vi "模拟器自动控制程序（轨迹跟踪）[2.1 alpha].vi"() -> ()   [LabVIEW 2012]
uses:
  <vilib>/Utility/error.llb/DialogType.ctl
  <vilib>/Platform/TimedLoop/XDataNode/timing_clust.ctl
  <vilib>/Platform/TimedLoop/XDataNode/nitl_modes.ctl
  <vilib>/Platform/TimedLoop/XDataNode/wakeup.ctl
  <vilib>/Instr/_visa.llb/VISA Configure Serial Port (Instr).vi
  <vilib>/DAQmx/create/channels.llb/DAQmx Create Channel (DO-Digital Output).vi
  <vilib>/Analysis/baseanly.llb/Real Dot Product.vi
  <vilib>/Analysis/Matrix/Numeric/Conversions/Array To Matrix - RA2.vi
  <vilib>/Utility/file.llb/Write To Spreadsheet File (DBL).vi
  <vilib>/Platform/TimedLoop/XDataNode/XDataNode.xnode
  <vilib>/Platform/TimedLoop/XDataNode/XDNodeRunTimeDep.lvlib
  <vilib>/Analysis/Matrix/NI_Matrix.lvlib
  <vilib>/vision/NI_Vision_Development_Module.lvlib
  <vilib>/Analysis/NI_AALBase.lvlib
panel:
  out "x/y":dbl
  out "Truster4":bool
  out "Truster 8":bool
  out "Truster  3":bool
  out "Truster 7":bool
  out "Truster 5":bool
  out "Truster  2":bool
  out "Truster 6":bool
  out "Truster1":bool
  out "定位点信息":T1(array[cluster]) {"Aspect Ratio" format="%.2f"; "Orientation" format="%.2f"; "Area" format="%.2f"; "Object Center"."Y" format="%.2f"; "Object Center"."X" format="%.2f"}
  out "alpha":dbl
  out "计时参数":dbl
  in  "卫星模拟器":enum32{"初始化", "运行监测"}(tab)
  out "读取缓冲区":string
  out "电流校正模式":bool
  out "软件使能":bool caption="软件使能(启动/停止)"
  out "电流校正中":bool caption="电流校正完成"
  out "E2PROM初始化结果":bool
  out "E2初始化完成":bool
  out "CRC校验和错误":bool
  out "串口通信错误":bool caption="串口通信故障"
  out "发送指令":string
  out "控制命令":string
  out "电机已启动":bool
  in  "采样率":i64=10
  in  "限制转速":dbl=500.0
  in  "ID号":u8=255 step=1 format="%#.0f"
  in  "最高转速":dbl=500.0
  in  "PWM周期":dbl=1599.0
  in  "最大力矩":dbl=2047.0
  in  "stop bits (10: 1 bit)":u16(ring)=10 caption="停止位" items=["1.0"=10, "1.5"=15, "2.0"=20]
  out "串口状态":bool
  in  "端口选择":refnum<visa-resource-name>="COM1"
  in  "波特率":u16(ring)=10 items=["   300", "   600", "   1200", "   2400", "   4800   ", "   9600", "   19200", "   38400", "   43000", "   56000", "   57600", "   115200"]
  in  "校验":enum16{"None", "Odd", "Even"}(ring)=enum."Even"
  in  "数据位":u16=8
  in  "打开":bool caption="stop"
  out "轨控信号":dbl
  in  "姿轨控开始":bool
  out "转速模式":bool
  out "转矩模式":bool
  out "故障":bool
  out "启停状态":bool
  in  "存储波形":bool
  in  "显示波形 停止显示":bool
  in  "开始记录":bool
  out "动量轮转矩":dbl format="%#_6f"
  out "动量轮转速":dbl format="%#_4f"
  out "X速率(cm/s)":dbl
  out "Y速率(cm/s)":dbl
  out "Y偏移量 (cm)":dbl
  out "X偏移量 (cm)":dbl
  out "相对偏角(deg)":dbl
  out "角速度(deg/s)":dbl
  out "设备ID":u8=255
  in  "模式选择":u16(ring)=1 items=["电流校正模式", "转矩模式", "转速模式", "开环测试模式"]
  in  "模式选择":bool
  in  "写指令字":dbl
  in  "清除故障":bool
  in  "停止电机":bool
  in  "启动电机":bool
  out "波形图":cluster{"转矩反馈":dbl, "转速反馈":dbl}(graph)
  in  "退出程序":bool caption="停止电机 2"
  in  "Floating":bool
  in  "缩放比例 (像素/cm)":dbl=4.099468
  in  "X中心校正":dbl
  in  "Y中心校正":dbl
  out "指令Y":dbl
  out "指令X":dbl
  out "指令角度":dbl
  out "alpha (deg)":dbl
  out "x >= y?":bool
  out "数值":dbl
  out "输出数组 6":dbl[](array[numeric])
  out "输出数组 7":dbl[](array[numeric])
  out "输出数组 10":dbl[](array[numeric])
  out "无符号字节数组 2":u8[](array[numeric])
  # "状态"
  # "设置"
  # "控制信号"
  # "参数确定"
  # "状态显示"
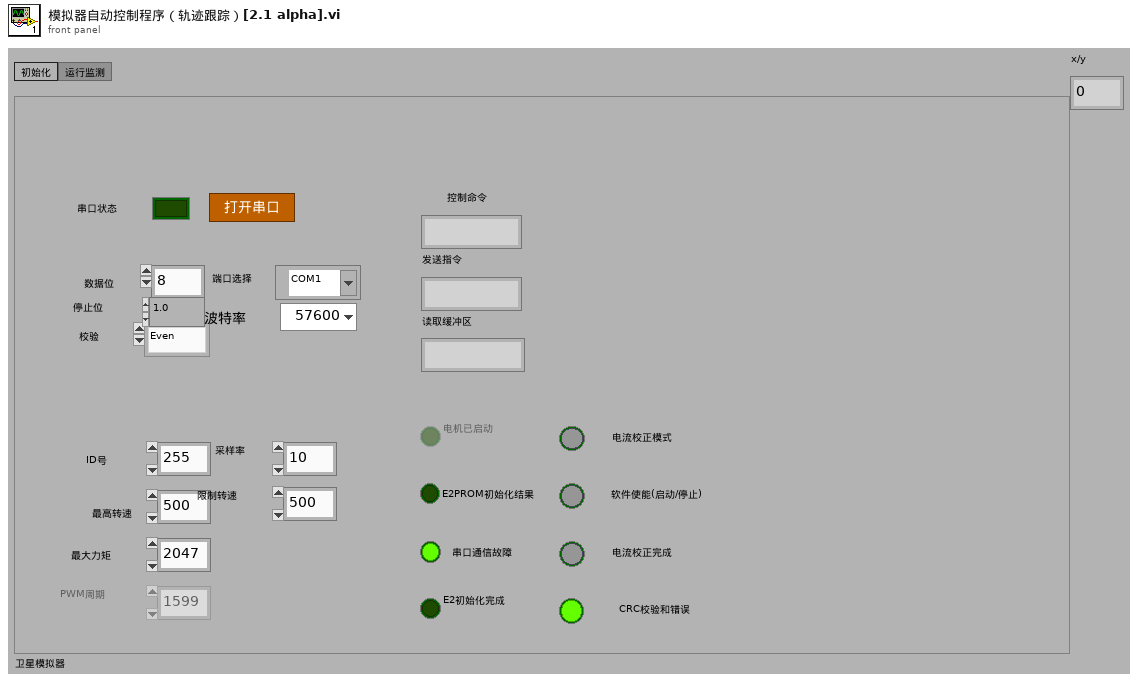
[diagram p1: front panel]
types:
  T1 = cluster{"Object Center":cluster{"X":sgl, "Y":sgl}, "Bounding Box":cluster{"X Left":i32, "Y Top":i32, "X Right":i32, "Y Bottom":i32}, "Area":sgl, "Orientation":sgl, "Aspect Ratio":sgl, "Nb Holes":i32}[]
  T2 = typedef "XDNodeRunTimeDep.lvlib/timing_clust.ctl" = cluster{"Expected End [f-1]":u64, "Actual End [f-1]":u64, "Finished Late? [f-1]":bool, "Expected End [i-1]":u64, "Actual End [i-1]":u64, "Finished Late? [i-1]":bool, "Expected Start [i]":u64, "Actual Start [i]":u64, "Expected Start [f]":u64, "Actual Start [f]":u64, "Source Name":string, "Structure Name":string, "Period":i64, "Deadline":i64, "Offset":i64, "Start":i64, "Priority":i32, "Timeout":i32, "Mode":T3, "Wakeup Reason":T4, "Error":errorcluster, "Source Type":string, "Secondary Source Type":string, "Global End Time":u64, "Global Start Time":u64, "Frame Duration":u64, "Iteration Duration":u64, "Assigned CPU":i32, "I/O Scan Engine Mode":u32}
  T3 = typedef "XDNodeRunTimeDep.lvlib/nitl_modes.ctl" = enum32{"No Change", "Process missed periods, maintain original phase", "Discard missed periods, maintain original phase", "Process missed periods, ignore original phase", "Discard missed periods, ignore original phase"}
  T4 = typedef "XDNodeRunTimeDep.lvlib/wakeup.ctl" = enum32{"Normal", "Aborted", "Asynchronous wakeup", "Timing source error", "Timed loop error", "Timeout"}
  T5 = cluster{"Objects":u16, "Threshold":i32, "Reject Border":bool, "Fill Holes":bool, "Min Object Size":bool, "Min Size":i32, "Max Object Size":bool, "Max Size":i32, "Show Search Area":bool, "Show Center":bool, "Show Bounding Box":bool}
  T6 = typedef "DialogType.ctl" = u16
  T7 = typedef "NI_Matrix.lvlib/RealMatrix.ctl" = dbl[][]
  T8 = typedef "IMAQ Image.ctl" = refnum<image>
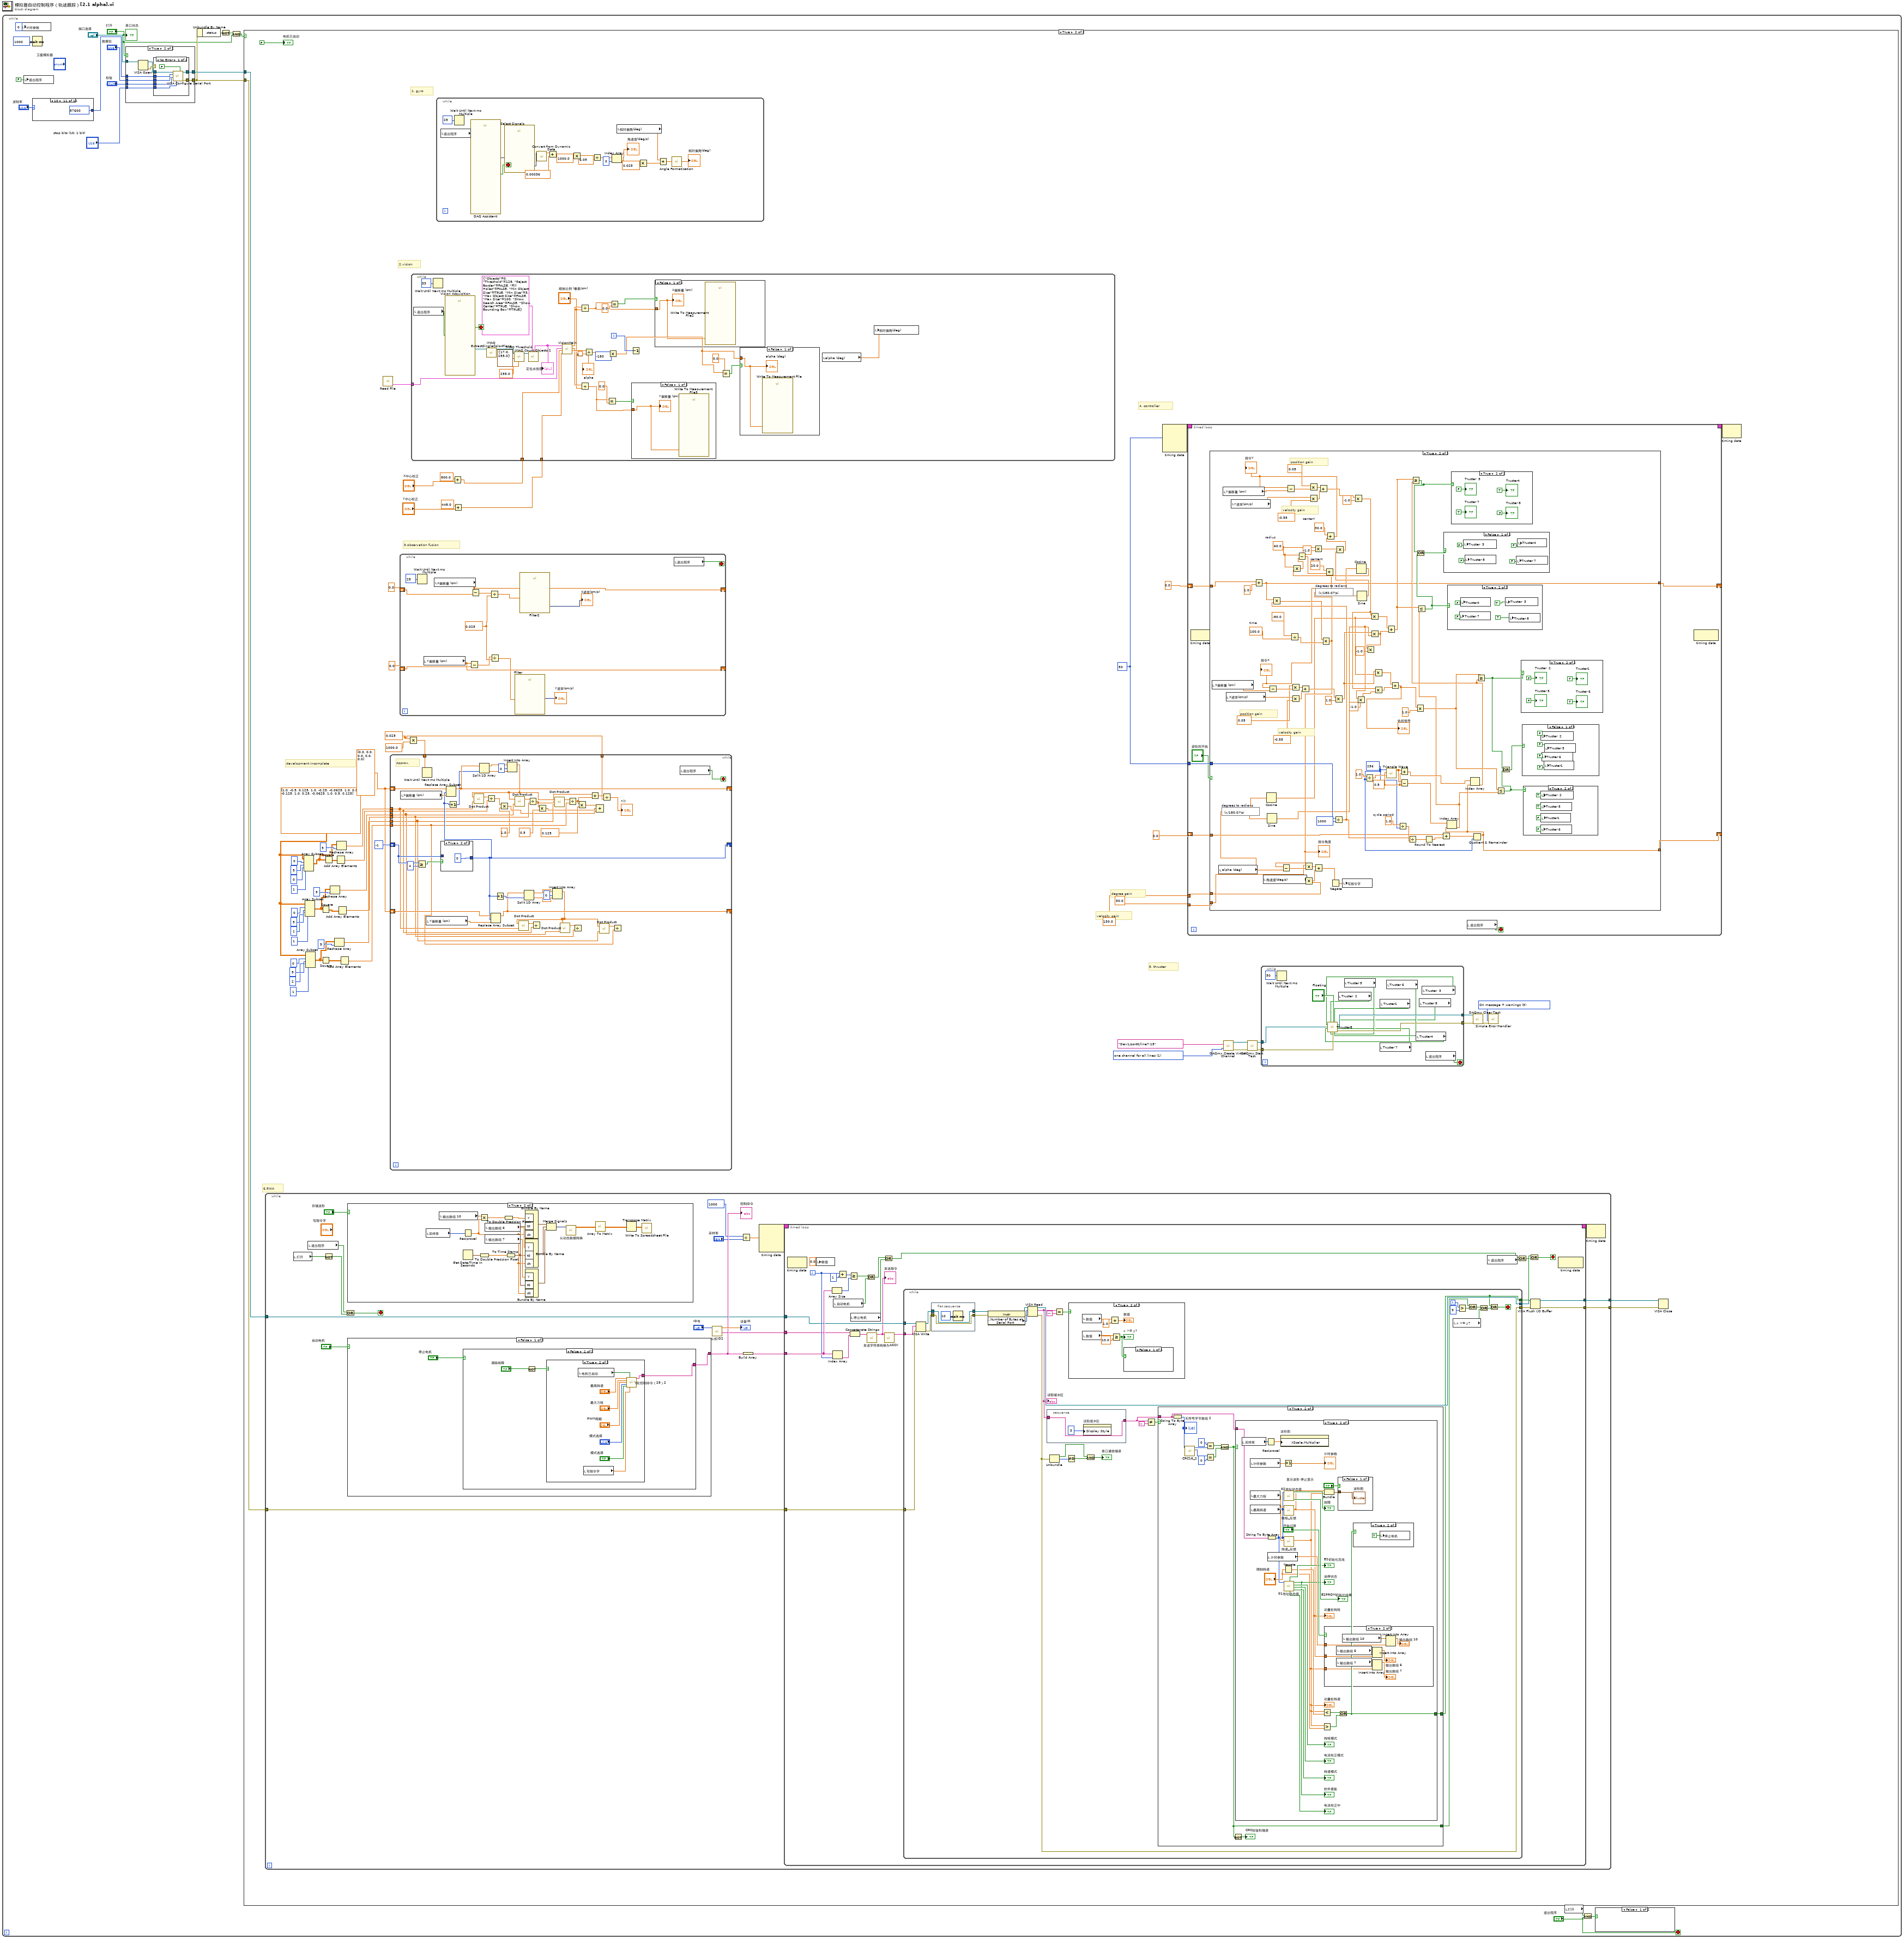
[diagram p0: block diagram]
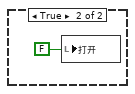
[diagram p2: hidden frame]
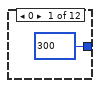
[diagram p5: hidden frame]
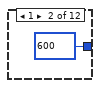
[diagram p6: hidden frame]
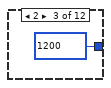
[diagram p7: hidden frame]
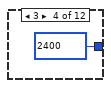
[diagram p8: hidden frame]
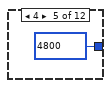
[diagram p9: hidden frame]
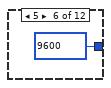
[diagram p10: hidden frame]
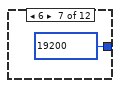
[diagram p11: hidden frame]
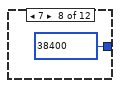
[diagram p12: hidden frame]
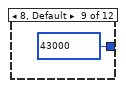
[diagram p13: hidden frame]
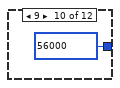
[diagram p14: hidden frame]
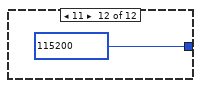
[diagram p15: hidden frame]
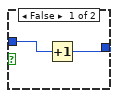
[diagram p17: hidden frame]
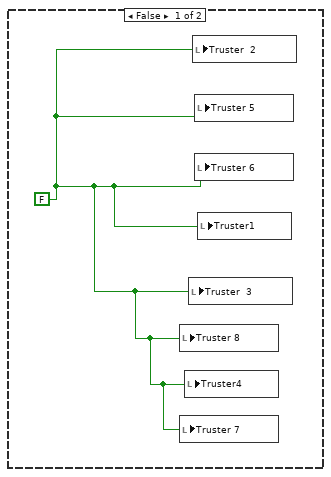
[diagram p18: hidden frame]
diagram:
  n1 = while {
    stop <- "退出程序" stop-if-true
    n2 = local write "计时参数"(0) -> ()
    n3 = local write "退出程序"(FALSE ("退出程序")) -> ()
    n4 = Wait (ms)(milliseconds to wait=u32 1000 ("等待时间（毫秒）")) -> ()  [unwired: 1 out]
    n5 = case shown="10" "波特率" {
      tunnel: [300 600 1200 2400 4800 9600 19200 38400 43000 56000 57600 115200] -> w17
      frame 0 {
      }
      frame 1 {
      }
      frame 2 {
      }
      frame 3 {
      }
      frame 4 {
      }
      frame 5 {
      }
      frame 6 {
      }
      frame 7 {
      }
      frame 8, Default {
      }
      frame 9 {
      }
      frame 10 {
      }
      frame 11 {
      }
    }
    n6 = case shown="True" "打开" {
      tunnel: w17 -> [_ w28]
      tunnel: "数据位" -> [_ w27]
      tunnel: "校验" -> [_ w26]
      tunnel: "端口选择" -> [_ w25]
      tunnel: [_ w22] -> w7
      tunnel: [_ w21] -> w6
      tunnel: "stop bits (10: 1 bit)" -> [_ w20]
      frame False {
      }
      frame True {
        n7 = VISA Open(VISA resource name=w25) -> (VISA resource name=w24:refnum<visa-resource-name>, error out=w23:errorcluster)  [unwired: 1 in, 3 out]
        n8 = case shown="No Error" w23 {
          tunnel: w28 -> [w36 _]
          tunnel: w27 -> [w35 _]
          tunnel: w26 -> [w34 _]
          tunnel: w24 -> [w33 _]
          tunnel: [w32 _] -> w22
          tunnel: [w31 _] -> w21
          tunnel: w20 -> [w30 _]
          frame No Error {
            n9 = call-poly "VISA Configure Serial Port"("VISA resource name"=w33, "Enable Termination\nChar (T)"=FALSE ("Enable Termination\nChar (T)"), "baud rate (9600)"=w36, "data bits (8)"=w35, "parity (0:none)"=w34, "stop bits (10: 1 bit)"=w30) -> ("VISA resource name out"=w32:refnum<visa-resource-name>, "error out"=w31:errorcluster)  [unwired: 2 in, 6 out]
          }
          frame Error {
          }
        }
      }
    }
    n10 = Unbundle By Name(w6) -> ("status"=w12:bool)
    n11 = Not(x=w12) -> (.not. x?=w11:bool)
    n12 = And(x=w11, y="打开") -> (x .and. y?=w8:bool)
    n13 = case shown="True" w8 {
      tunnel: w7 -> [_ w109]
      tunnel: w6 -> [_ w108]
      frame False {
      }
      frame True {
        w49 = 0.025
        w65 = dbl[][] [[1.0, -0.5, 0.125], [1.0, -0.25, -0.0625], [1.0, 0.0, -0.125], [1.0, 0.25, -0.0625], [1.0, 0.5, 0.125]]
        w52 = dbl[] [0.0, 0.0, 0.0, 0.0, 0.0]
        w89 = 1 items=["one channel for each line", "one channel for all lines"] ("line grouping")
        w91 = T6 3 items=["no dialog", "OK message", "continue or stop message", "OK message + warnings", "continue/stop + warnings"] ("type of dialog (OK msg:1)")
        w85 = 50
        # "development incomplete"
        # "5. thruster"
        # "6.RWA"
        # "4. controller"
        # "3.observation fusion"
        # "2.vision"
        # "1. gyro"
        # "velocity gain"
        # "degree gain"
        n14 = while {
          tunnel: [w379] -> w111
          tunnel: [w378] -> w110
          tunnel: w109 -> [w377]
          tunnel: w108 -> [w376]
          stop <- w372 stop-if-true
          n15 = local read "打开"() -> (w375:bool)
          n16 = local read "退出程序"() -> (w374:bool)
          n17 = Not(x=w375) -> (.not. x?=w373:bool)
          n18 = Or(x=w374, y=w373) -> (x .or. y?=w372:bool)
          n19 = case shown="True" "存储波形" {
            frame False {
            }
            frame True {
              n20 = local read "采样率"() -> (w404:i64)
              n21 = local read "输出数组 10"() -> (w397:dbl[])
              n22 = Reciprocal(x=w404) -> (1/x=w399:dbl)
              n23 = Get Date/Time In Seconds() -> (seconds since 1Jan1904=w408:timestamp)
              n24 = Multiply(x=w397, y=w399) -> (x*y=w398:dbl[])
              n25 = To Double Precision Float(number=w408) -> (double precision float=w407:dbl)
              n26 = local read "输出数组 6"() -> (w406:dbl[])
              n27 = local read "输出数组 7"() -> (w405:dbl[])
              n28 = To Double Precision Float(number=w398) -> (double precision float=w396:dbl[])
              n29 = To Time Stamp(1:w407) -> (0:w400:timestamp)
              n30 = Bundle By Name("Y"=w396, "t0"=w400, "dt"=w399) -> (w401:waveform(dbl))  [unwired: 1 out]
              n31 = Bundle By Name("Y"=w406, "t0"=w400, "dt"=w399) -> (w402:waveform(dbl))  [unwired: 1 out]
              n32 = Bundle By Name("Y"=w405, "t0"=w400, "dt"=w399) -> (w403:waveform(dbl))  [unwired: 1 out]
              n33 = Merge Signals(w401, w402, w403) -> (w395:dynamicdata)
              n34 = call "从动态数据转换"("Dynamic Data Type"=w395) -> ("Array"=w394:dbl[][])  [unwired: 3 in]
              n35 = call-poly <vilib>:"Array To Matrix.vi"("Real 2D Array"=w394) -> ("Real Matrix"=w393:T7)
              n36 = Transpose Matrix(1:w393) -> (0:w392:T7)
              n37 = call-poly <vilib>:"Write To Spreadsheet File.vi"("2D data"=w392) -> ()  [unwired: 7 in, 1 out]
            }
          }
          n38 = case shown="False" "启动电机" {
            tunnel: [w535 w562] -> w388
            frame False {
              n39 = case shown="False" "停止电机" {
                tunnel: [w536 w555] -> w535
                frame False {
                  n40 = Not(x="清除故障") -> (.not. x?=w537:bool)
                  n41 = case shown="True" w537 {
                    tunnel: [w539 w548] -> w536
                    frame False {
                      n42 = call <vilib>:"Space Constant.vi"() -> ("String"=w543:string)
                      n43 = Concatenate Strings(w543, "05" ("字符串"), w543, "23" ("字符串"), w543, "01" ("字符串")) -> (w539:string)
                    }
                    frame True {
                      n44 = local read "电机已启动"() -> (w545:bool)
                      n45 = local read "写指令字"() -> (w544:dbl)
                      n46 = call "飞轮控制命令（29）2.vi"("最高转速"="最高转速", "电机启动控制指令"=w545, "力矩最大值"="最大力矩", "pwmperiod"="PWM周期", "模式选择 3"="模式选择", "模式选择 4"="模式选择", "写指令字"=w544) -> ("字符串"=w548:string)  [unwired: 8 in]
                    }
                  }
                }
                frame True {
                  n47 = local write "电机已启动"(FALSE) -> ()
                  n48 = local write "启动电机"(FALSE ("停止电机")) -> ()
                  n49 = local write "停止电机"(FALSE ("停止电机")) -> ()
                  n50 = call <vilib>:"Space Constant.vi"() -> ("String"=w559:string)
                  n51 = Concatenate Strings(w559, "05" ("字符串"), w559, "22" ("字符串"), w559, "00" ("字符串")) -> (w555:string)
                }
              }
            }
            frame True {
              n52 = local write "电机已启动"(TRUE) -> ()
              n53 = local write "启动电机"(FALSE) -> ()
              n54 = call <vilib>:"Space Constant.vi"() -> ("String"=w566:string)
              n55 = Concatenate Strings(w566, "05" ("字符串"), w566, "22" ("字符串"), w566, "01" ("字符串")) -> (w562:string)
            }
          }
          "控制命令" <- w388
          n56 = call "从机ID2.vi"("ID号"="ID号") -> ("字符串"=w380:string, "设备ID"=→"设备ID":dbl)  [unwired: 9 in]
          n57 = Divide(x=i64 1000 ("Period"), y="采样率") -> (x/y=w384:dbl)
          n58 = Build Array(w388) -> (w385:string[])
          n59 = node-c288(w384) -> (w387:T2)  [unwired: 3 in]
          n60 = timed-loop {
            timing: w387 -> [_]
            timing-out: [_] -> w386
            tunnel: w385 -> [w429]
            tunnel: w380 -> [w425]
            tunnel: [w422] -> w379
            tunnel: [w421] -> w378
            tunnel: w377 -> [w420]
            tunnel: w376 -> [w419]
            i -> [w428]
            stop <- w409 stop-if-true
            n61 = node-c288() -> ()  [unwired: 1 in, 1 out]
            n62 = local write "数值"(0.0 ("y")) -> ()
            n63 = Array Size(array=w429) -> (size(s)=w433:i32)
            n64 = Index Array(array=w429, index=w428) -> (element=w432:string)
            n65 = local read "启动电机"() -> (w416:bool)
            n66 = Add(x=w428, y=1) -> (x+y=w434:i32)
            n67 = Greater Or Equal?(x=w434, y=w433) -> (x >= y?=w417:bool)
            n68 = Concatenate Strings(w425, w432) -> (w431:string)
            n69 = local read "停止电机"() -> (w415:bool)
            n70 = Or(x=w417, y=w416) -> (x .or. y?=w414:bool)
            n71 = call "发送字符串.vi"("字符串"=w431) -> ("连接的字符串 2"=w418:string)  [unwired: 10 in]
            "发送指令" <- w418
            n72 = Or(x=w414, y=w415) -> (x .or. y?=w412:bool)
            n73 = call "转换为ASCII.vi"("字符串"=w418) -> ("字符串 2"=w430:string)  [unwired: 10 in]
            n74 = while {
              tunnel: [w462] -> w423
              tunnel: [w451] -> w424
              tunnel: w430 -> [w456]
              tunnel: w420 -> [w437]
              tunnel: w419 -> [w436]
              tunnel: [w435] -> w411
              i -> [w461]
              stop <- w444 stop-if-true
              n75 = VISA Write(VISA resource name=w437, write buffer=w456, error in (no error)=w436) -> (VISA resource name out=w442:refnum<visa-resource-name>, error out=w439:errorcluster)  [unwired: 1 out]
              n76 = flat-sequence {
                tunnel: w442 -> [w468]
                tunnel: [w468] -> w441
                tunnel: [w467] -> w440
                tunnel: w439 -> [w467]
                frame #0 {
                  n77 = Wait (ms)(milliseconds to wait=i64 10 ("Period")) -> ()  [unwired: 1 out]
                }
              }
              n78 = property class="Instr"(reference=w441, error in=w440) -> (reference out=w464:refnum<visa-resource-name>, error out=w463:errorcluster, "Serial Settings:Number of Bytes at Serial Port"=w465:u32)
              n79 = VISA Read(VISA resource name=w464, byte count=w465, error in (no error)=w463) -> (VISA resource name out=w462:refnum<visa-resource-name>, read buffer=w455:string, error out=w451:errorcluster)  [unwired: 1 out]
              "读取缓冲区" <- w455
              n80 = stacked-sequence {
                tunnel: [w519] -> w454
                tunnel: w455 -> [w519]
                frame #0 {
                  n81 = property on="读取缓冲区" class="Str"("Display Style"=u32 3 ("显示样式")) -> ()  [unwired: 2 in, 2 out]
                }
              }
              n82 = Unbundle(w451) -> ("status"=w448:bool, "code"=w450:i32)  [unwired: 1 out]
              n83 = Equal?(x=w455, y="") -> (x = y?=w458:bool)
              n84 = Not Equal To 0?(x=w450) -> (x != 0?=w449:bool)
              n85 = case shown="True" w458 {
                frame False {
                  n86 = local write "数值"(0.0 ("数值")) -> ()
                }
                frame True {
                  n87 = local read "数值"() -> (w521:dbl)
                  n88 = local read "数值"() -> (w526:dbl)
                  n89 = Add(x=w521, y=1.0) -> (x+y=→"数值":dbl)
                  n90 = Greater Or Equal?(x=w526, y=10.0) -> (x >= y?=w524:bool)
                  "x >= y?" <- w524
                  n91 = case shown="False" w524 {
                    frame False {
                    }
                    frame True {
                      n92 = local write "打开"(FALSE) -> ()
                    }
                  }
                }
              }
              n93 = And(x=w448, y=w449) -> (x .and. y?=→"串口通信错误":bool)
              n94 = Not Equal?(x=w454, y="") -> (x != y?=w443:bool)
              n95 = case shown="True" w443 {
                tunnel: w454 -> [_ w479]
                tunnel: [_ w473] -> w452
                tunnel: [_ w474] -> w435
                frame False {
                }
                frame True {
                  n96 = String To Byte Array(string=w479) -> (unsigned byte array=w469:u8[])
                  "无符号字节数组 2" <- w469
                  n97 = call "CRC16_2.vi"("buf"=w469) -> ("CRCHi"=w470:u8, "CRCLo"=w471:u8)  [unwired: 9 in]
                  n98 = Equal?(x=u8 0, y=w471) -> (x = y?=w475:bool)
                  n99 = Equal?(x=w470, y=u8 0) -> (x = y?=w476:bool)
                  n100 = And(x=w475, y=w476) -> (x .and. y?=w473:bool)
                  n101 = Not(x=w473) -> (.not. x?=→"CRC校验和错误":bool)
                  n102 = case shown="True" w473 {
                    tunnel: w479 -> [_ w506]
                    tunnel: [_ w480] -> w474
                    frame False {
                    }
                    frame True {
                      n103 = local read "采样率"() -> (w504:i64)
                      n104 = local read "计时参数"() -> (w501:dbl)
                      n105 = local read "最大力矩"() -> (w489:dbl)
                      n106 = local read "最高转速"() -> (w487:dbl)
                      n107 = Reciprocal(x=w504) -> (1/x=w503:dbl)
                      n108 = String To Byte Array(string=w506) -> (unsigned byte array=w486:u8[])
                      n109 = local read "计时参数"() -> (w498:dbl)
                      n110 = property on="波形图" class="WFChart (strict)"("XScale.Multiplier"=w503) -> ()  [unwired: 2 in, 2 out]
                      n111 = Increment(x=w501) -> (x+1=→"计时参数":dbl)
                      n112 = Negate(x="限制转速") -> (-x=w485:dbl)
                      n113 = call "02地址状态值.vi"("unsigned byte array"=w486) -> ("E2初始化失败"=→"E2PROM初始化结果":bool, "故障"=→"故障":bool)  [unwired: 9 in]
                      n114 = call "转矩_反馈.vi"("unsigned byte array"=w486, "最大转矩"=w489) -> ("转矩反馈"=w488:dbl)  [unwired: 9 in]
                      "动量轮转矩" <- w488
                      n115 = call "转速_反馈.vi"("最高转速"=w487, "unsigned byte array"=w486) -> ("转速反馈"=w484:dbl)  [unwired: 9 in]
                      "动量轮转速" <- w484
                      n116 = call "01地址状态值.vi"("unsigned byte array"=w486) -> ("E2初始化完成"=→"E2初始化完成":bool, "电流校正完成"=→"电流校正中":bool, "启停状态"=→"软件使能" →"启停状态":bool, "转矩模式"=→"转矩模式":bool, "电流校正"=→"电流校正模式":bool, "转速模式"=→"转速模式":bool)  [unwired: 4 in]
                      n117 = Less?(x=w484, y=w485) -> (x < y?=w481:bool)
                      n118 = Greater?(x=w484, y="限制转速") -> (0:w482:bool)
                      n119 = Bundle("转矩反馈"=w488, "转速反馈"=w484) -> (w505:cluster{"转矩反馈":dbl, "转速反馈":dbl})  [unwired: 1 out]
                      n120 = case shown="True" "开始记录" {
                        tunnel: w488 -> [_ w510]
                        tunnel: w484 -> [_ w509]
                        tunnel: w498 -> [_ w508]
                        frame False {
                        }
                        frame True {
                          n121 = local read "输出数组 6"() -> (w515:dbl[])
                          n122 = local read "输出数组 7"() -> (w513:dbl[])
                          n123 = local read "输出数组 10"() -> (w511:dbl[])
                          n124 = Insert Into Array(array=w515, new element=w510) -> (→"输出数组 6":dbl[])  [unwired: 1 in]
                          n125 = Insert Into Array(array=w513, new element=w509) -> (→"输出数组 7":dbl[])  [unwired: 1 in]
                          n126 = Insert Into Array(array=w511, new element=w508) -> (→"输出数组 10":dbl[])  [unwired: 1 in]
                        }
                      }
                      n127 = case shown="False" "显示波形 停止显示" {
                        tunnel: w505 -> [w517 _]
                        frame False {
                          "波形图" <- w517
                        }
                        frame True {
                        }
                      }
                      n128 = Or(x=w481, y=w482) -> (x .or. y?=w480:bool)
                      n129 = case shown="True" w480 {
                        frame False {
                        }
                        frame True {
                          n130 = local write "停止电机"(TRUE ("停止电机")) -> ()
                        }
                      }
                    }
                  }
                }
              }
              n131 = local read "x >= y?"() -> (w446:bool)
              n132 = Greater?(x=w461, y=9) -> (0:w438:bool)
              n133 = Or(x=w452, y=w438) -> (x .or. y?=w457:bool)
              n134 = Or(x=w457, y=w446) -> (x .or. y?=w445:bool)
              n135 = Or(x=w435, y=w445) -> (x .or. y?=w444:bool)
            }
            n136 = local read "退出程序"() -> (w413:bool)
            n137 = Or(x=w412, y=w413) -> (x .or. y?=w410:bool)
            n138 = Or(x=w411, y=w410) -> (x .or. y?=w409:bool)
            n139 = VISA Flush I/O Buffer(VISA resource name=w423, error in (no error)=w424) -> (VISA resource name out=w422:refnum<visa-resource-name>, error out=w421:errorcluster)  [unwired: 1 out]
            n140 = node-c288() -> ()  [unwired: 1 in, 1 out]
          }
          n141 = node-c288(w386) -> ()  [unwired: 1 out]
        }
        n142 = Array Subset(array=w65, index (row)=0 ("index"), length (row)=5 ("length"), index (col)=0 ("index"), length (col)=1 ("length")) -> (w63:dbl[][])
        n143 = Array Subset(array=w65, index (row)=0 ("index"), length (row)=5 ("length"), index (col)=1 ("index"), length (col)=1 ("length")) -> (w59:dbl[][])
        n144 = Array Subset(array=w65, index (row)=0 ("index"), length (row)=5 ("length"), index (col)=2 ("index"), length (col)=1 ("length")) -> (w55:dbl[][])
        n145 = Square(x=w59) -> (x^2=w67:dbl[][])
        n146 = Square(x=w55) -> (x^2=w66:dbl[][])
        n147 = Square(x=w63) -> (x^2=w68:dbl[][])
        n148 = Reshape Array(w59, 5 ("dimension size")) -> (w58:dbl[])
        n149 = Reshape Array(w55, 5 ("dimension size")) -> (w54:dbl[])
        n150 = Add Array Elements(numeric array=w68) -> (sum=w61:dbl)
        n151 = Reshape Array(w63, 5 ("dimension size")) -> (w62:dbl[])
        n152 = Add Array Elements(numeric array=w67) -> (sum=w57:dbl)
        n153 = Add Array Elements(numeric array=w66) -> (sum=w53:dbl)
        n154 = call "Read File.vi"() -> ("Objects"=w106:T1)  [unwired: 1 in, 1 out]
        n155 = while {
          shift-right: [w365] -> _
          shift-left: 0.0 ("X偏移量 (cm)") -> [w364]
          shift-right: [w362] -> _
          shift-left: 0.0 ("Y偏移量 (cm)") -> [w361]
          stop <- w370 stop-if-true
          w363 = 0.025 ("y")
          n156 = Wait Until Next ms Multiple(millisecond multiple=u32 25) -> ()  [unwired: 1 out]
          n157 = local read "Y偏移量 (cm)"() -> (w362:dbl)
          n158 = local read "X偏移量 (cm)"() -> (w365:dbl)
          n159 = Subtract(x=w362, y=w361) -> (x-y=w367:dbl)
          n160 = Subtract(x=w365, y=w364) -> (x-y=w368:dbl)
          n161 = Divide(x=w368, y=w363) -> (x/y=w359:dbl)
          n162 = Divide(x=w367, y=w363) -> (x/y=w360:dbl)
          n163 = call "Filter"("Signal"=w360) -> ("Filtered Signal"=→"Y速率(cm/s)":dynamicdata)  [unwired: 9 in, 1 out]
          n164 = call "Filter2"("Signal"=w359) -> ("Filtered Signal"=→"X速率(cm/s)":dynamicdata)  [unwired: 9 in, 1 out]
          n165 = local read "退出程序"() -> (w370:bool)
        }
        n166 = Multiply(x=w49, y=1000.0) -> (x*y=w50:dbl)
        n167 = while {
          shift-right: [w149] -> _
          shift-left: w52 -> [w157]
          shift-right: [w141] -> _
          shift-left: -1 -> [w153]
          tunnel: w62 -> [w134]
          tunnel: w61 -> [w133]
          tunnel: w58 -> [w132]
          tunnel: w57 -> [w130]
          tunnel: w54 -> [w128]
          tunnel: w53 -> [w127]
          shift-right: [w139] -> _
          shift-left: w52 -> [w142]
          tunnel: w50 -> [w115]
          tunnel: w49 -> [w114]
          stop <- w158 stop-if-true
          # "Approx."
          n168 = local read "X偏移量 (cm)"() -> (w156:dbl)
          n169 = Greater Or Equal?(x=w153, y=4) -> (x >= y?=w154:bool)
          n170 = Wait Until Next ms Multiple(millisecond multiple=w115) -> ()  [unwired: 1 out]
          n171 = local read "Y偏移量 (cm)"() -> (w143:dbl)
          n172 = case shown="True" w154 {
            tunnel: [w159 0] -> w141
            tunnel: w153 -> [w160 _]
            frame False {
              n173 = Increment(x=w160) -> (x+1=w159:i32)
            }
            frame True {
            }
          }
          n174 = Replace Array Subset(array=w157, new element=w156, index=w141) -> (w149:dbl[])
          n175 = Increment(x=w141) -> (x+1=w148:i32)
          n176 = Split 1D Array(array=w149, index=w148) -> (first subarray=w146:dbl[], second subarray=w147:dbl[])
          n177 = Replace Array Subset(array=w142, new element=w143, index=w141) -> (w139:dbl[])
          n178 = Increment(x=w141) -> (x+1=w140:i32)
          n179 = Insert Into Array(array=w146, index=0, new element=w147) -> (w144:dbl[])
          n180 = call-poly <vilib>:"Dot Product.vi"("Y Vector"=w134, "X Vector"=w144) -> ("X * Y"=w152:dbl)  [unwired: 1 out]
          n181 = Divide(x=w152, y=w133) -> (x/y=w125:dbl)
          n182 = Multiply(x=w125, y=1.0) -> (x*y=w119:dbl)
          n183 = call-poly <vilib>:"Dot Product.vi"("Y Vector"=w132, "X Vector"=w144) -> ("X * Y"=w151:dbl)  [unwired: 1 out]
          n184 = Split 1D Array(array=w139, index=w140) -> (first subarray=w138:dbl[], second subarray=w137:dbl[])
          n185 = Divide(x=w151, y=w130) -> (x/y=w118:dbl)
          n186 = Multiply(x=w118, y=0.5) -> (x*y=w120:dbl)
          n187 = Insert Into Array(array=w138, index=0, new element=w137) -> (w129:dbl[])
          n188 = call-poly <vilib>:"Dot Product.vi"("Y Vector"=w134, "X Vector"=w129) -> ("X * Y"=w135:dbl)  [unwired: 1 out]
          n189 = Divide(x=w135, y=w133) -> ()  [unwired: 1 out]
          n190 = call-poly <vilib>:"Dot Product.vi"("Y Vector"=w128, "X Vector"=w144) -> ("X * Y"=w150:dbl)  [unwired: 1 out]
          n191 = call-poly <vilib>:"Dot Product.vi"("Y Vector"=w132, "X Vector"=w129) -> ("X * Y"=w131:dbl)  [unwired: 1 out]
          n192 = Divide(x=w150, y=w127) -> (x/y=w117:dbl)
          n193 = Divide(x=w131, y=w130) -> ()  [unwired: 1 out]
          n194 = Multiply(x=w117, y=0.125) -> (x*y=w121:dbl)
          n195 = Add(x=w118, y=w117) -> (x+y=w116:dbl)
          n196 = Compound Arithmetic op=ADD(w121, w120, w119) -> ()  [unwired: 1 out]
          n197 = call-poly <vilib>:"Dot Product.vi"("Y Vector"=w128, "X Vector"=w129) -> ("X * Y"=w126:dbl)  [unwired: 1 out]
          n198 = Divide(x=w116, y=w114) -> (x/y=→"x/y":dbl)
          n199 = Divide(x=w126, y=w127) -> ()  [unwired: 1 out]
          n200 = local read "退出程序"() -> (w158:bool)
        }
        n201 = while {
          stop <- w358 stop-if-true
          n202 = local read "退出程序"() -> (w345:bool)
          n203 = Wait Until Next ms Multiple(millisecond multiple=u32 25 ("y")) -> ()  [unwired: 1 out]
          n204 = call "DAQ Assistant"("stop (F)"=w345) -> ("data"=w343:dynamicdata, "stopped"=w358:bool)  [unwired: 15 in, 2 out]
          n205 = call "Select Signals"("Signals"=w343) -> ("Signal Out"=w344:dynamicdata)  [unwired: 9 in, 1 out]
          n206 = call "Convert from Dynamic Data"("Dynamic Data Type"=w344) -> ("Array"=w349:dbl[])  [unwired: 3 in]
          n207 = Add(x=w349, y=0.00036) -> (x+y=w347:dbl[])
          n208 = Multiply(x=w347, y=1000.0) -> (x*y=w357:dbl[])
          n209 = Divide(x=w357, y=6.09) -> (x/y=w351:dbl[])
          n210 = Index Array(array=w351, index=0) -> (element=w341:dbl)
          "角速度(deg/s)" <- w341
          n211 = local read "相对偏角(deg)"() -> (w346:dbl)
          n212 = Multiply(x=w341, y=0.025) -> (x*y=w352:dbl)
          n213 = Add(x=w346, y=w352) -> (x+y=w342:dbl)
          n214 = call "Angle Formatization.vi"("Alpha"=w342) -> ("Alpha Formatized"=→"相对偏角(deg)":dbl)
        }
        n215 = Add(x=800.0 ("c_x"), y="X中心校正") -> (x+y=w103:dbl)
        n216 = Add(x=448.0 ("c_y"), y="Y中心校正") -> (x+y=w100:dbl)
        n217 = while {
          tunnel: w106 -> [w311]
          tunnel: w100 -> [w305]
          tunnel: w103 -> [w304]
          i -> [w307]
          stop <- w321 stop-if-true
          n218 = local read "退出程序"() -> (w313:bool)
          n219 = Wait Until Next ms Multiple(millisecond multiple=u32 33 ("y")) -> ()  [unwired: 1 out]
          n220 = call "Vision Acquisition"("Stop (F)"=w313) -> ("Image Out"=w317:T8, "Stopped"=w321:bool)  [unwired: 24 in, 1 out]
          n221 = call "IMAQ ExtractSingleColorPlane"("Image Src"=w317) -> ("Image Dst Out"=w302:T8)  [unwired: 9 in, 1 out]
          n222 = call "IMAQ Threshold"("Replace Value"=sgl 255.0 ("replace value"), "Range"=cluster{"lower value":sgl, "upper value":sgl} {"lower value"=17.0, "upper value"=255.0} ("threshold"), "Image Src"=w302) -> ("Image Dst Out"=w318:T8)  [unwired: 7 in, 1 out]
          n223 = call "IMAQ Count Objects 2"("Settings"=T5 {"Objects"=0, "Threshold"=128, "Reject Border"=FALSE, "Fill Holes"=FALSE, "Min Object Size"=TRUE, "Min Size"=3, "Max Object Size"=FALSE, "Max Size"=100, "Show Search Area"=FALSE, "Show Center"=TRUE, "Show Bounding Box"=TRUE}, "Image"=w318) -> ("Objects"=w312:T1)  [unwired: 5 in, 4 out]
          "定位点信息" <- w312
          n224 = call "VisionMain.vi"("Y Center"=w305, "X Center"=w304, "Original Plots"=w311, "Plots Captured"=w312) -> ("alpha"=w310:dbl, "dy"=w309:dbl, "dx"=w308:dbl)  [unwired: 5 in]
          "alpha" <- w310
          n225 = Divide(x=w308, y="缩放比例 (像素/cm)") -> (x/y=w296:dbl)
          n226 = Divide(x=w309, y="缩放比例 (像素/cm)") -> (x/y=w293:dbl)
          n227 = Divide(x=w310, y=3.141592653589793) -> (x/y=w315:dbl)
          n228 = Equal?(x=w293, y=0.0) -> (x = y?=w294:bool)
          n229 = Multiply(x=w315, y=-180) -> (x*y=w299:dbl)
          n230 = Equal?(x=w296, y=0.0) -> (x = y?=w297:bool)
          n231 = Decrement(x=w307) -> ()  [unwired: 1 out]
          n232 = case shown="False" w294 {
            tunnel: w293 -> [w322 _]
            frame False {
              n233 = call "Write To Measurement File3"("Signals"=w322) -> ()  [unwired: 16 in, 3 out]
              "Y偏移量 (cm)" <- w322
            }
            frame True {
            }
          }
          n234 = case shown="False" w297 {
            tunnel: w296 -> [w323 _]
            frame False {
              n235 = call "Write To Measurement File2"("Signals"=w323) -> ()  [unwired: 16 in, 3 out]
              "X偏移量 (cm)" <- w323
            }
            frame True {
            }
          }
          n236 = Equal?(x=w299, y=0.0) -> (x = y?=w300:bool)
          n237 = case shown="False" w300 {
            tunnel: w299 -> [w324 _]
            frame False {
              n238 = call "Write To Measurement File"("Signals"=w324) -> ()  [unwired: 16 in, 3 out]
              "alpha (deg)" <- w324
            }
            frame True {
            }
          }
          n239 = local read "alpha (deg)"() -> (w292:dbl)
          n240 = local write "相对偏角(deg)"(w292) -> ()
        }
        n241 = node-c288(w85) -> (w87:T2)  [unwired: 3 in]
        n242 = timed-loop {
          tunnel: 30.0 ("degree gain") -> [w170]
          tunnel: 130.0 ("angular velocity gain") -> [w169]
          shift-right: [w168] -> _
          shift-left: 0.0 -> [w167]
          tunnel: w85 -> [w166]
          timing: w87 -> [_]
          timing-out: [_] -> w86
          shift-right: [w163] -> _
          shift-left: 0.0 -> [w162]
          stop <- w165 stop-if-true
          n243 = node-c288() -> ()  [unwired: 1 in, 1 out]
          n244 = case shown="True" "姿轨控开始" {
            tunnel: w170 -> [_ w258]
            tunnel: w169 -> [_ w257]
            tunnel: [_ w229] -> w168
            tunnel: w167 -> [_ w228]
            tunnel: w166 -> [_ w227]
            tunnel: [_ w192] -> w163
            tunnel: w162 -> [_ w209]
            frame False {
              w171 = FALSE ("Truster 6")
              n245 = local write "Truster 8"(w171) -> ()
              n246 = local write "Truster 7"(w171) -> ()
              n247 = local write "Truster4"(w171) -> ()
              n248 = local write "Truster  3"(w171) -> ()
              n249 = local write "Truster  2"(w171) -> ()
              n250 = local write "Truster 5"(w171) -> ()
              n251 = local write "Truster 6"(w171) -> ()
              n252 = local write "Truster1"(w171) -> ()
            }
            frame True {
              w185 = 20.0  # centerX
              w189 = 30.0  # centerY
              w191 = 60.0  # radius
              w207 = 100.0  # time
              w233 = 256 ("samples")
              w240 = 1.0  # cycle period
              w244 = 0.5 ("amplitude")
              # "position gain"
              # "velocity gain"
              # "velocity gain"
              # "position gain"
              n253 = local read "X偏移量 (cm)"() -> (w251:dbl)
              n254 = local read "alpha (deg)"() -> (w172:dbl)
              n255 = expression code="(x/180.0)*pi" "degrees to radians"(w172) -> (w175:dbl)
              n256 = local read "Y偏移量 (cm)"() -> (w220:dbl)
              n257 = local read "X速率(cm/s)"() -> (w249:dbl)
              n258 = local read "Y速率(cm/s)"() -> (w218:dbl)
              n259 = Add(x=w209, y=1.0) -> (x+y=w192:dbl)
              n260 = local read "角速度(deg/s)"() -> (w253:dbl)
              n261 = Cosine(x=w175) -> (cos(x)=w173:dbl)
              n262 = Sine(x=w175) -> (sin(x)=w174:dbl)
              n263 = Divide(x=-90.0 ("time"), y=w207) -> (x/y=w205:dbl)
              n264 = Multiply(x=w249, y=-0.55) -> (x*y=w247:dbl)
              n265 = Multiply(x=w253, y=w257) -> (x*y=w256:dbl)
              n266 = Multiply(x=w218, y=-0.55) -> (x*y=w222:dbl)
              n267 = Multiply(x=w191, y=-1.0) -> (x*y=w188:dbl)
              n268 = Divide(x=w227, y=u32 1000) -> (x/y=w206:dbl)
              n269 = Multiply(x=w192, y=w206) -> (x*y=w193:dbl)
              n270 = Multiply(x=w193, y=w205) -> (x*y=w176:dbl)
              "指令角度" <- w176
              n271 = Subtract(x=w176, y=w172) -> (x-y=w260:dbl)
              n272 = Multiply(x=w258, y=w260) -> (x*y=w259:dbl)
              n273 = Add(x=w259, y=w256) -> (x+y=w255:dbl)
              n274 = expression code="(x/180.0)*pi" "degrees to radians"(w176) -> (w204:dbl)
              n275 = Negate(x=w255) -> (-x=w254:dbl)
              n276 = local write "写指令字"(w254) -> ()
              n277 = Cosine(x=w204) -> (cos(x)=w195:dbl)
              n278 = Multiply(x=w191, y=w195) -> (x*y=w203:dbl)
              n279 = Subtract(x=w191, y=w203) -> (x-y=w184:dbl)
              n280 = Add(x=w185, y=w184) -> (x+y=w183:dbl)
              "指令X" <- w183
              n281 = Subtract(x=w183, y=w251) -> (x-y=w252:dbl)
              n282 = Multiply(x=0.05 ("degree gain"), y=w252) -> (x*y=w246:dbl)
              n283 = Add(x=w246, y=w247) -> (x+y=w225:dbl)
              n284 = Multiply(x=w225, y=1.0) -> (x*y=w196:dbl)
              n285 = Multiply(x=w174, y=-1.0) -> (x*y=w179:dbl)
              n286 = Sine(x=w204) -> (sin(x)=w178:dbl)
              n287 = Multiply(x=w188, y=w178) -> (x*y=w187:dbl)
              n288 = Add(x=w189, y=w187) -> (x+y=w186:dbl)
              "指令Y" <- w186
              n289 = Subtract(x=w186, y=w220) -> (x-y=w224:dbl)
              n290 = Multiply(x=0.05 ("degree gain"), y=w224) -> (x*y=w221:dbl)
              n291 = Add(x=w221, y=w222) -> (x+y=w211:dbl)
              n292 = Multiply(x=w211, y=-1.0) -> (x*y=w194:dbl)
              n293 = Divide(x=1.0 ("amplitude"), y=w233) -> (x/y=w241:dbl)
              n294 = Multiply(x=w194, y=w173) -> (x*y=w201:dbl)
              n295 = Multiply(x=w196, y=w174) -> (x*y=w200:dbl)
              n296 = Multiply(x=w200, y=-1.0) -> ()  [unwired: 1 out]
              n297 = Multiply(x=w196, y=w173) -> (x*y=w198:dbl)
              n298 = Multiply(x=w194, y=w179) -> (x*y=w197:dbl)
              n299 = call <vilib>:"Triangle Wave.vi"("samples"=w233, "amplitude"=w244, "frequency"=w241) -> ("triangle wave"=w245:dbl[])  [unwired: 2 in, 2 out]
              n300 = Add(x=w201, y=w200) -> (x+y=w199:dbl)
              n301 = Add(x=w198, y=w197) -> (x+y=w182:dbl)
              "轨控信号" <- w182
              n302 = Divide(x=w240, y=w233) -> (x/y=w239:dbl)
              n303 = Add(x=w245, y=w244) -> (x+y=w237:dbl[])
              n304 = Subtract(x=w245, y=w244) -> (x-y=w236:dbl[])
              n305 = Divide(x=w206, y=w239) -> (x/y=w238:dbl)
              n306 = Multiply(x=w182, y=1.0) -> (x*y=w180:dbl)
              n307 = Round To Nearest(number=w238) -> (nearest integer value=w235:dbl)
              n308 = Add(x=w228, y=w235) -> (x+y=w234:dbl)
              n309 = Quotient & Remainder(x=w234, y=w233) -> (x-y*floor(x/y)=w229:dbl)  [unwired: 1 out]
              n310 = Index Array(array=w236, index=w229) -> (element=w216:dbl)
              n311 = Less Or Equal?(x=w199, y=w216) -> (x <= y?=w214:bool)
              n312 = case shown="True" w214 {
                frame False {
                }
                frame True {
                  n313 = local write "Truster 7"(FALSE ("Truster 6")) -> ()
                  n314 = local write "Truster4"(FALSE ("Truster 6")) -> ()
                  n315 = local write "Truster  3"(TRUE ("Truster 6")) -> ()
                  n316 = local write "Truster 8"(TRUE ("Truster 6")) -> ()
                }
              }
              n317 = Index Array(array=w237, index=w229) -> (element=w217:dbl)
              n318 = Greater Or Equal?(x=w199, y=w217) -> (x >= y?=w215:bool)
              n319 = Or(x=w215, y=w214) -> (x .or. y?=w213:bool)
              n320 = case shown="False" w213 {
                frame False {
                  n321 = local write "Truster  3"(FALSE ("Truster 6")) -> ()
                  n322 = local write "Truster 8"(FALSE ("Truster 6")) -> ()
                  n323 = local write "Truster 7"(FALSE ("Truster 6")) -> ()
                  n324 = local write "Truster4"(FALSE ("Truster 6")) -> ()
                }
                frame True {
                }
              }
              n325 = case shown="True" w215 {
                frame False {
                }
                frame True {
                  "Truster4" <- TRUE ("Truster 6")
                  "Truster 8" <- FALSE ("Truster 6")
                  "Truster  3" <- FALSE ("Truster 6")
                  "Truster 7" <- TRUE ("Truster 6")
                }
              }
              n326 = Greater Or Equal?(x=w180, y=w217) -> (x >= y?=w232:bool)
              n327 = Less Or Equal?(x=w180, y=w216) -> (x <= y?=w231:bool)
              n328 = Or(x=w232, y=w231) -> (x .or. y?=w230:bool)
              n329 = case shown="True" w232 {
                frame False {
                }
                frame True {
                  "Truster1" <- TRUE ("Truster 6")
                  "Truster 6" <- TRUE ("Truster 6")
                  "Truster  2" <- FALSE ("Truster 6")
                  "Truster 5" <- FALSE ("Truster 6")
                }
              }
              n330 = case shown="False" w230 {
                frame False {
                  n331 = local write "Truster  2"(FALSE ("Truster 6")) -> ()
                  n332 = local write "Truster 6"(FALSE ("Truster 6")) -> ()
                  n333 = local write "Truster1"(FALSE ("Truster 6")) -> ()
                  n334 = local write "Truster 5"(FALSE ("Truster 6")) -> ()
                }
                frame True {
                }
              }
              n335 = case shown="True" w231 {
                frame False {
                }
                frame True {
                  n336 = local write "Truster  2"(TRUE ("Truster 6")) -> ()
                  n337 = local write "Truster 5"(TRUE ("Truster 6")) -> ()
                  n338 = local write "Truster 6"(FALSE ("Truster 6")) -> ()
                  n339 = local write "Truster1"(FALSE ("Truster 6")) -> ()
                }
              }
            }
          }
          n340 = local read "退出程序"() -> (w165:bool)
          n341 = node-c288() -> ()  [unwired: 1 in, 1 out]
        }
        n342 = call-poly <vilib>:"DAQmx Create Virtual Channel.vi"("lines"=tag "Dev1/port0/line7:15" ("Lines"), "line grouping"=w89) -> ("task out"=w94:refnum<k21>, "error out"=w93:errorcluster)  [unwired: 12 in]
        n343 = call <vilib>:"DAQmx Start Task.vi"("task/channels in"=w94, "error in"=w93) -> ("task out"=w96:refnum<k21>, "error out"=w99:errorcluster)  [unwired: 12 in]
        n344 = while {
          tunnel: w99 -> [w335]
          tunnel: [w336] -> w98
          tunnel: w96 -> [w338]
          tunnel: [w337] -> w95
          stop <- w339 stop-if-true
          n345 = Wait Until Next ms Multiple(millisecond multiple=u32 50) -> ()  [unwired: 1 out]
          n346 = local read "Truster  2"() -> (w332:bool)
          n347 = local read "Truster 5"() -> (w333:bool)
          n348 = local read "Truster 7"() -> (w325:bool)
          n349 = local read "Truster1"() -> (w331:bool)
          n350 = local read "Truster 6"() -> (w330:bool)
          n351 = local read "Truster4"() -> (w326:bool)
          n352 = local read "Truster 8"() -> (w327:bool)
          n353 = local read "Truster  3"() -> (w328:bool)
          n354 = call "Thruster8.vi"("Thruster 2"=w332, "Truster1"=w331, "Floating"="Floating", "Thruster 3"=w328, "Thruster 8"=w327, "task in"=w338, "Thruster 4"=w326, "Thruster 7"=w325, "Thruster 5"=w333, "error in"=w335, "Thruster 6"=w330) -> ("task out"=w337:refnum<k21>, "error out"=w336:errorcluster)  [unwired: 3 in]
          n355 = local read "退出程序"() -> (w339:bool)
        }
        n356 = call <vilib>:"DAQmx Clear Task.vi"("task in"=w95, "error in"=w98) -> ("error out"=w97:errorcluster)  [unwired: 13 in]
        n357 = call <vilib>:"Simple Error Handler.vi"("type of dialog (OK msg:1)"=w91, "error in (no error)"=w97) -> ()  [unwired: 3 in, 5 out]
        n358 = VISA Close(VISA resource name=w111, error in (no error)=w110) -> ()  [unwired: 1 out]
        n359 = node-c288(w86) -> ()  [unwired: 1 out]
        "电机已启动" <- FALSE
      }
    }
    n360 = local read "打开"() -> (w3:bool)
    n361 = And(x=w3, y="退出程序") -> (x .and. y?=w1:bool)
    n362 = case shown="False" w1 {
      frame False {
      }
      frame True {
        n363 = local write "打开"(FALSE ("打开")) -> ()
      }
    }
    "串口状态" <- "打开"
  }
